vi "GetDiagramUIDs.vi"(6 "error in":errorcluster, 9 "DiagramDisable in":refnum<class "DiagramDisable.lvclass">) -> (0 "error out":errorcluster, 3 "DiagramDisable out":refnum<class "DiagramDisable.lvclass">, 4 "diagrams":i32[](array[numeric]))   [LabVIEW 2014, in "DiagramDisable.lvclass"]
uses:
  DiagramDisable.lvclass
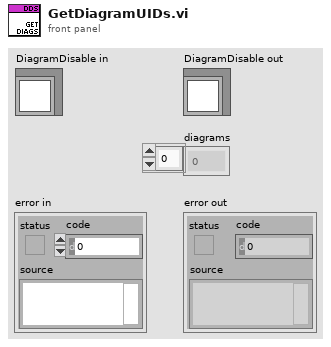
[diagram p1: front panel]
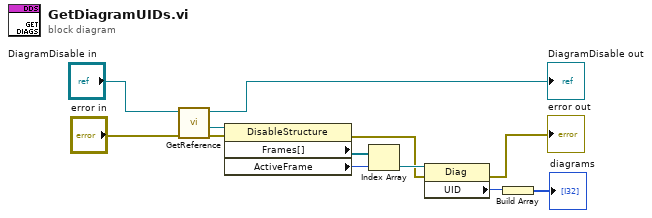
[diagram p0: block diagram]
diagram:
  n1 = call "GetReference.vi"("error in"="error in", "DiagramDisable in"="DiagramDisable in") -> ("error out"=w10:errorcluster, "DDS reference"=w11:refnum<vi>, "DiagramDisable out"=→"DiagramDisable out":refnum<class "DiagramDisable.lvclass">)  [unwired: 7 in]
  n2 = property class="DisableStructure"(reference=w11, error in=w10) -> (error out=w6:errorcluster, "Frames[]"=w8:refnum<vi>[], "ActiveFrame"=w9:i16)  [unwired: 1 out]
  n3 = Index Array(array=w8, index=w9) -> (element=w7:refnum<vi>)
  n4 = property class="Diag"(reference=w7, error in=w6) -> (error out=→"error out":errorcluster, "UID"=w2:i32)  [unwired: 1 out]
  n5 = Build Array(w2) -> (→"diagrams":i32[])
